vi "CaseStructureToErrorCS.vi"(8 "error in (no error)":errorcluster, 10 "reference":refnum<vi>) -> (0 "error out":errorcluster)   [LabVIEW 2014]
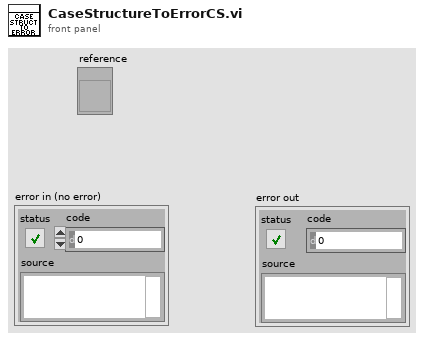
[diagram p1: front panel]
types:
  T1 = typedef "LVBoundsTypeDef.ctl" = cluster{"Width":u32, "Height":u32}
  T2 = typedef "LVPositionTypeDef.ctl" = cluster{"Left":i32, "Top":i32}
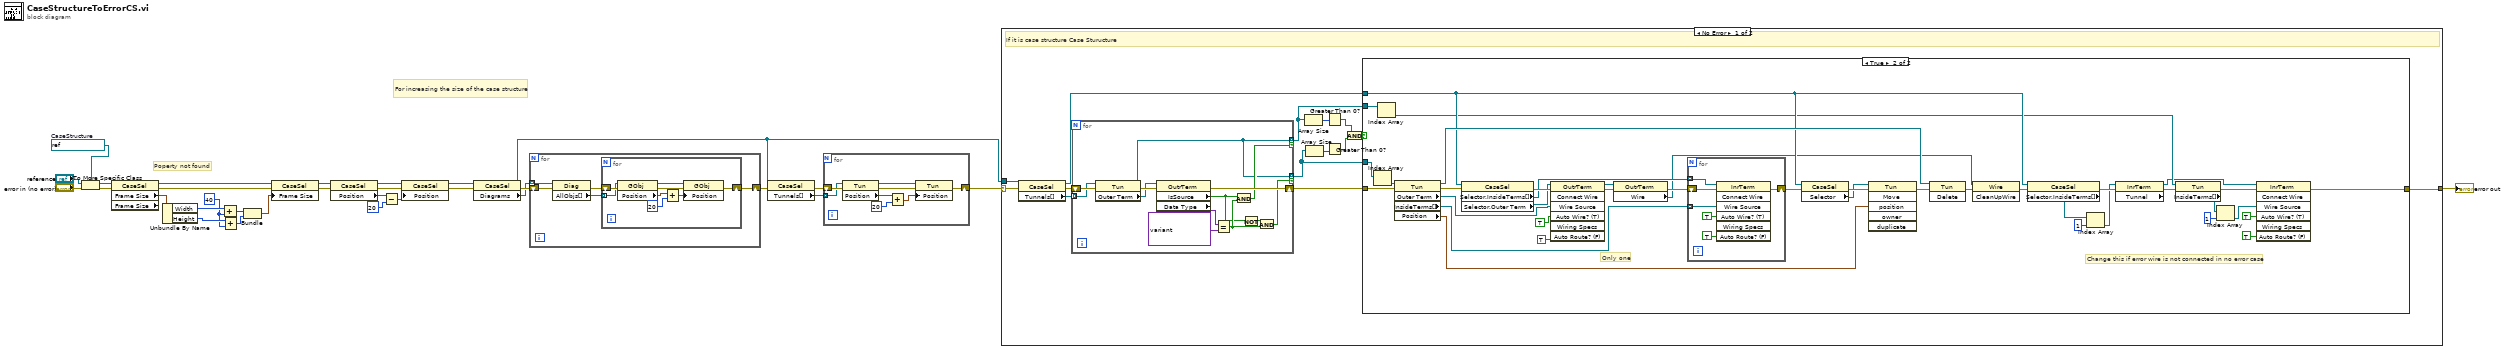
[diagram p0: block diagram]
diagram:
  w15 = u32 40 ("y")
  w28 = refnum<vi> refnum  # CaseStructure
  # "Poperty not found"
  # "For increasing the size of the case structure"
  n1 = To More Specific Class(target class=w28, reference="reference", error in="error in (no error)") -> (specific class reference=w26:refnum<vi>, error out=w29:errorcluster)
  n2 = property class="CaseSel" props=["Frame Size", "Frame Size"](reference=w26, error in=w29) -> (reference out=w22:refnum<vi>, error out=w23:errorcluster, "Frame Size"=w21:T1)  [unwired: 1 out]
  n3 = Unbundle By Name(w21) -> ("Width"=w20:u32, "Height"=w17:u32)
  n4 = Add(x=w20, y=w15) -> (x+y=w19:u32)
  n5 = Add(x=w17, y=w15) -> (x+y=w18:u32)
  n6 = Bundle(w19, w18) -> (w16:cluster{u32, u32})  [unwired: 1 in]
  n7 = property class="CaseSel"(reference=w22, error in=w23, "Frame Size"=w16) -> (reference out=w13:refnum<vi>, error out=w14:errorcluster)
  n8 = property class="CaseSel"(reference=w13, error in=w14) -> (reference out=w10:refnum<vi>, error out=w12:errorcluster, "Position"=w8:T2)
  n9 = Subtract(x=w8, y=u32 20) -> (x-y=w6:cluster{"Left":u32, "Top":u32})
  n10 = property class="CaseSel"(reference=w10, error in=w12, "Position"=w6) -> (reference out=w9:refnum<vi>, error out=w11:errorcluster)
  n11 = property class="CaseSel"(reference=w9, error in=w11) -> (reference out=w4:refnum<vi>, error out=w25:errorcluster, "Diagrams"=w24:refnum<vi>[])
  n12 = for {
    shift-right: [w33] -> w5
    shift-left: w25 -> [w36]
    tunnel: w24 -> [w35] mode=indexing
    n13 = property class="Diag"(reference=w35, error in=w36) -> (error out=w34:errorcluster, "AllObjs[]"=w32:refnum<vi>[])  [unwired: 1 out]
    n14 = for {
      tunnel: w32 -> [w43] mode=indexing
      shift-right: [w41] -> w33
      shift-left: w34 -> [w44]
      n15 = property class="GObj"(reference=w43, error in=w44) -> (reference out=w40:refnum<vi>, error out=w42:errorcluster, "Position"=w39:T2)
      n16 = Add(x=w39, y=u32 20) -> (x+y=w38:cluster{"Left":u32, "Top":u32})
      n17 = property class="GObj"(reference=w40, error in=w42, "Position"=w38) -> (error out=w41:errorcluster)  [unwired: 1 out]
    }
  }
  n18 = property class="CaseSel"(reference=w4, error in=w5) -> (error out=w3:errorcluster, "Tunnels[]"=w1:refnum<vi>[])  [unwired: 1 out]
  n19 = for {
    shift-right: [w49] -> w2
    shift-left: w3 -> [w52]
    tunnel: w1 -> [w51] mode=indexing
    n20 = property class="Tun"(reference=w51, error in=w52) -> (reference out=w48:refnum<vi>, error out=w50:errorcluster, "Position"=w47:T2)
    n21 = Add(x=w47, y=u32 20) -> (x+y=w46:cluster{"Left":u32, "Top":u32})
    n22 = property class="Tun"(reference=w48, error in=w50, "Position"=w46) -> (error out=w49:errorcluster)  [unwired: 1 out]
  }
  n23 = case shown="No Error" w2 {
    selector: w2 -> [w66 w126]
    tunnel: [w61 w126] -> w31
    tunnel: w4 -> [w65 _]
    frame No Error {
      # "If it is case structure Case Sturucture"
      n24 = property class="CaseSel"(reference=w65, error in=w66) -> (reference out=w53:refnum<vi>, error out=w64:errorcluster, "Tunnels[]"=w63:refnum<vi>[])
      n25 = for {
        shift-right: [w122] -> w62
        shift-left: w64 -> [w125]
        tunnel: w63 -> [w124] mode=indexing
        tunnel: [w114] -> w54 mode=indexing if=w116
        tunnel: [w114] -> w55 mode=indexing if=w115
        n26 = property class="Tun"(reference=w124, error in=w125) -> (reference out=w114:refnum<vi>, error out=w123:errorcluster, "Outer Term"=w121:refnum<vi>)
        n27 = property class="OutrTerm"(reference=w121, error in=w123) -> (error out=w122:errorcluster, "IsSource"=w117:bool, "Data Type"=w120:variant)  [unwired: 1 out]
        n28 = Equal?(x=w120, y=variant(errorcluster {"status"=FALSE, "code"=0, "source"=""}) ("variant")) -> (x = y?=w119:bool)
        n29 = And(x=w117, y=w119) -> (x .and. y?=w116:bool)
        n30 = Not(x=w117) -> (.not. x?=w118:bool)
        n31 = And(x=w118, y=w119) -> (x .and. y?=w115:bool)
      }
      n32 = Array Size(array=w54) -> (size(s)=w60:i32)
      n33 = Array Size(array=w55) -> (size(s)=w59:i32)
      n34 = Greater Than 0?(x=w60) -> (x > 0?=w58:bool)
      n35 = Greater Than 0?(x=w59) -> (x > 0?=w57:bool)
      n36 = And(x=w58, y=w57) -> (x .and. y?=w56:bool)
      n37 = case shown="True" w56 {
        tunnel: [w67 w86] -> w61
        tunnel: w62 -> [w67 w105]
        tunnel: w55 -> [_ w104]
        tunnel: w54 -> [_ w87]
        tunnel: w53 -> [_ w91]
        frame False {
          # "No error wire inside case structure"
        }
        frame True {
          # "Only one"
          # "Change this if error wire is not connected in no error case"
          n38 = Index Array(array=w104) -> (element=w103:refnum<vi>)  [unwired: 1 in]
          n39 = Index Array(array=w87) -> (element=w85:refnum<vi>)  [unwired: 1 in]
          n40 = property class="Tun"(reference=w103, error in=w105) -> (reference out=w95:refnum<vi>, error out=w74:errorcluster, "Outer Term"=w73:refnum<vi>, "InsideTerms[]"=w98:refnum<vi>[], "Position"=w97:T2)
          n41 = property class="CaseSel"(reference=w91, error in=w74) -> (error out=w106:errorcluster, "Selector.InsideTerms[]"=w100:refnum<vi>[], "Selector.Outer Term"=w102:refnum<vi>)  [unwired: 1 out]
          n42 = invoke class="OutrTerm" method="Connect Wire"(reference=w102, error in=w106, "Wire Source"=w73, "Auto Wire? (T)"=TRUE, "Auto Route? (F)"=TRUE) -> (reference out=w72:refnum<vi>, error out=w101:errorcluster)  [unwired: 2 in, 5 out]
          n43 = property class="OutrTerm"(reference=w72, error in=w101) -> (error out=w71:errorcluster, "Wire"=w68:refnum<vi>)  [unwired: 1 out]
          n44 = for {
            tunnel: w100 -> [w111] mode=indexing
            shift-right: [w110] -> w94
            shift-left: w71 -> [w112]
            tunnel: w98 -> [w109] mode=indexing
            n45 = invoke class="InrTerm" method="Connect Wire"(reference=w111, error in=w112, "Wire Source"=w109, "Auto Wire? (T)"=TRUE, "Auto Route? (F)"=TRUE) -> (error out=w110:errorcluster)  [unwired: 2 in, 6 out]
          }
          n46 = property class="CaseSel"(reference=w91, error in=w94) -> (error out=w93:errorcluster, "Selector"=w92:refnum<vi>)  [unwired: 1 out]
          n47 = invoke class="Tun" method="Move"(reference=w92, error in=w93, "position"=w97) -> (error out=w96:errorcluster)  [unwired: 3 in, 5 out]
          n48 = invoke class="Tun" method="Delete"(reference=w95, error in=w96) -> (error out=w70:errorcluster)  [unwired: 1 in, 2 out]
          n49 = invoke class="Wire" method="CleanUpWire"(reference=w68, error in=w70) -> (error out=w69:errorcluster)  [unwired: 1 in, 2 out]
          n50 = property class="CaseSel"(reference=w91, error in=w69) -> (error out=w89:errorcluster, "Selector.InsideTerms[]"=w90:refnum<vi>[])  [unwired: 1 out]
          n51 = Index Array(array=w90, index=1) -> (element=w88:refnum<vi>)
          n52 = property class="InrTerm" props=["Tunnel"](reference=w88, error in=w89) -> (reference out=w81:refnum<vi>, error out=w78:errorcluster)  [unwired: 1 out]
          n53 = property class="Tun"(reference=w85, error in=w78) -> (error out=w77:errorcluster, "InsideTerms[]"=w80:refnum<vi>[])  [unwired: 1 out]
          n54 = Index Array(array=w80, index=1) -> (element=w79:refnum<vi>)
          n55 = invoke class="InrTerm" method="Connect Wire"(reference=w81, error in=w77, "Wire Source"=w79, "Auto Wire? (T)"=TRUE, "Auto Route? (F)"=TRUE) -> (error out=w86:errorcluster)  [unwired: 2 in, 6 out]
        }
      }
    }
    frame Error {
      # "Discard if selection is not a case structure"
    }
  }
  "error out" <- w31
